vi "ABSTimeString_To_TimeStamp.vi"(8 "error in (no error)":errorcluster, 10 "is UTC (F)":bool=TRUE, 11 "Time String":string="2020-04-07T08:16:02.648352") -> (0 "error out":errorcluster, 3 "Time Stamp":timestamp)   [LabVIEW 2018]
uses:
  <vilib>/Utility/miscctls.llb/LVDateTimeRec.ctl
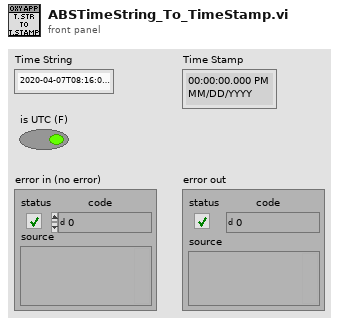
[diagram p1: front panel]
types:
  T1 = typedef "LVDateTimeRec.ctl" = cluster{"fractional second":dbl, "second":i32, "minute":i32, "hour":i32, "day of month":i32, "month":i32, "year":i32, "day of week":i32, "day of year":i32, "DST":i32}
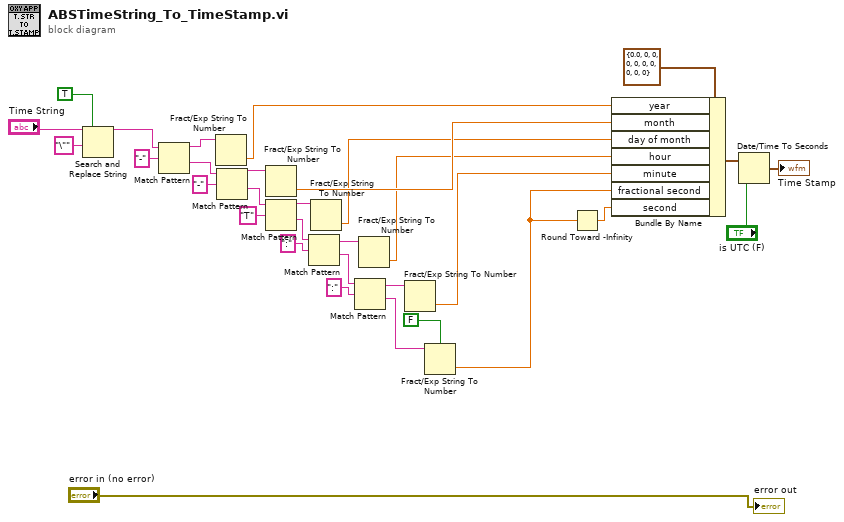
[diagram p0: block diagram]
diagram:
  n1 = Search and Replace String(replace all?=TRUE ("replace all? (F)"), input string="Time String", search string="\"") -> (result string=w1:string)  [unwired: 5 in, 3 out]
  n2 = Match Pattern(string=w1, regular expression="-") -> (before substring=w28:string, after substring=w30:string)  [unwired: 1 in, 2 out]
  n3 = Fract/Exp String To Number(string=w28) -> (number=w23:dbl)  [unwired: 3 in, 1 out]
  n4 = Match Pattern(string=w30, regular expression="-") -> (before substring=w26:string, after substring=w29:string)  [unwired: 1 in, 2 out]
  n5 = Fract/Exp String To Number(string=w26) -> (number=w22:dbl)  [unwired: 3 in, 1 out]
  n6 = Match Pattern(string=w29, regular expression="T") -> (before substring=w24:string, after substring=w20:string)  [unwired: 1 in, 2 out]
  n7 = Match Pattern(string=w20, regular expression=":") -> (before substring=w18:string, after substring=w14:string)  [unwired: 1 in, 2 out]
  n8 = Fract/Exp String To Number(string=w24) -> (number=w21:dbl)  [unwired: 3 in, 1 out]
  n9 = Match Pattern(string=w14, regular expression=":") -> (before substring=w16:string, after substring=w10:string)  [unwired: 1 in, 2 out]
  n10 = Fract/Exp String To Number(string=w18) -> (number=w17:dbl)  [unwired: 3 in, 1 out]
  n11 = Fract/Exp String To Number(string=w16) -> (number=w8:dbl)  [unwired: 3 in, 1 out]
  n12 = Fract/Exp String To Number(use system decimal point (T)=FALSE, string=w10) -> (number=w7:dbl)  [unwired: 2 in, 1 out]
  n13 = Round Toward -Infinity(1:w7) -> (0:w6:dbl)
  n14 = Bundle By Name(cluster=T1 {"fractional second"=0.0, "second"=0, "minute"=0, "hour"=0, "day of month"=0, "month"=0, "year"=0, "day of week"=0, "day of year"=0, "DST"=0} ("date time rec"), "year"=w23, "month"=w22, "day of month"=w21, "hour"=w17, "minute"=w8, "fractional second"=w7, "second"=w6) -> (w13:T1)
  n15 = Date/Time To Seconds(1:"is UTC (F)", 2:w13) -> (0:→"Time Stamp":timestamp)
  "error out" <- "error in (no error)"
